vi "fetch_and_translate_trigger.vi"(8 "error in (no error)":errorcluster, 11 "DAQ_DL090211Scaffold in":refnum<class "DAQ_DL090211Scaffold.lvclass">) -> (0 "error out":errorcluster, 1 "sender TLC type":T1=enum."ImagingMode", 2 "trigger":T2, 3 "DAQ_DL090211Scaffold out":refnum<class "DAQ_DL090211Scaffold.lvclass">)   [LabVIEW 2010, in "DAQ_DL090211Scaffold.lvclass"]
uses:
  DAQ_DL090211Scaffold.lvclass
  internal_trigger_enum.ctl
  common/enumerations/top-level_component_type_enum.ctl
  GenericDAQ/GenericDAQ/trigger_enum.ctl
  GenericDAQ/GenericDAQ/GenericDAQ.lvclass
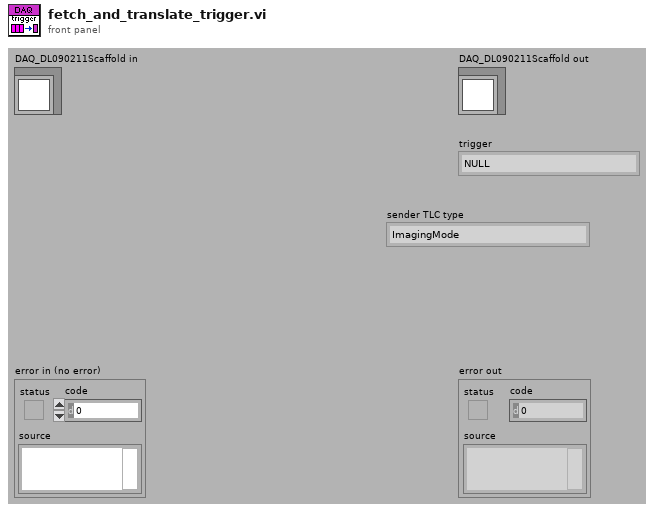
[diagram p1: front panel]
types:
  T1 = typedef "top-level_component_type_enum.ctl" = enum16{"undefined", "ImagingMode", "ScanHead", "DAQ", "ImageAssembler", "Display", "DataCollection", "Analyser", "Stimulator", "ExperimentController", "Instrument", "Stage"}
  T2 = typedef "DAQ_DL090211Scaffold.lvclass/internal_trigger_enum.ctl" = enum16{"NULL", "initialise", "terminate", "start", "stop", "read", "attach observer", "detach observer", "reset"}
  T3 = typedef "GenericDAQ.lvclass/trigger_enum.ctl" = enum16{"NULL", "read"}
  T4 = typedef "GenericToplevelComponent.lvclass/common_trigger_enum.ctl" = enum16{"NULL", "initialise", "terminate", "fetch command", "fetch data", "attach observer", "register as observer", "detach observer", "acknowledge", "start", "stop", "sweep started", "sweep finished", "experiment started", "experiment stopped"}
  T5 = typedef "trigger_type_enum.ctl" = enum8{"external", "internal", "common"}
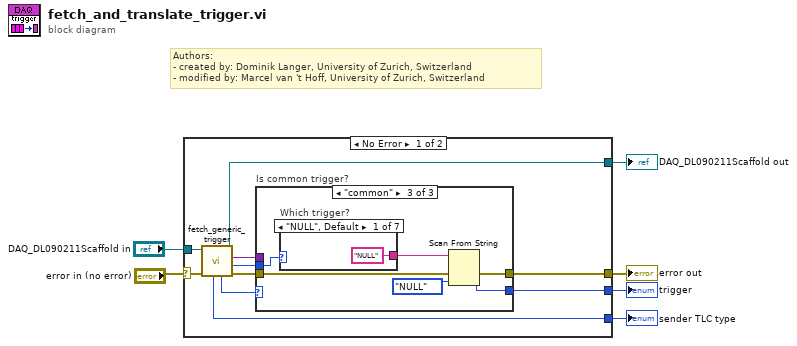
[diagram p0: block diagram]
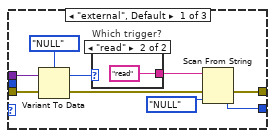
[diagram p2: hidden frame]
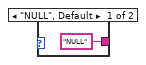
[diagram p3: hidden frame]
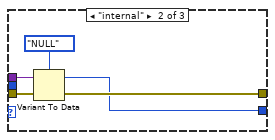
[diagram p4: hidden frame]
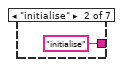
[diagram p5: hidden frame]
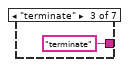
[diagram p6: hidden frame]
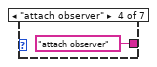
[diagram p7: hidden frame]
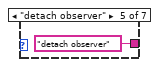
[diagram p8: hidden frame]
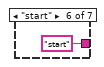
[diagram p9: hidden frame]
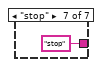
[diagram p10: hidden frame]
diagram:
  # "Authors: \n- created by: Dominik Langer, University of Zurich, Switzerland\n- modified by: Marcel van 't Hoff, University of Zurich, Switzerland"
  n1 = case shown="No Error" "error in (no error)" {
    selector: "error in (no error)" -> [w16 w47]
    tunnel: [w8 w47] -> w5
    tunnel: [w14 w46] -> w3
    tunnel: "DAQ_DL090211Scaffold in" -> [w15 w46]
    tunnel: [w7 _] -> w1
    tunnel: [w9 _] -> w2
    frame No Error {
      n2 = call-dynamic "fetch_generic_trigger.vi"("error in (no error)"=w16, "GenericToplevelComponent in"=w15) -> ("error out"=w12:errorcluster, "common trigger"=w10:T4, "trigger"=w11:variant, "GenericToplevelComponent out"=w14:refnum<class "DAQ_DL090211Scaffold.lvclass">, "trigger type"=w13:T5, "sender TLC type"=w9:T1)  [unwired: 3 in, 1 out]
      n3 = case "Is common trigger?" shown="\"common\"" w13 {
        tunnel: w12 -> [w25 w31 w36]
        tunnel: w11 -> [w24 w32 _]
        tunnel: w10 -> [_ _ w38]
        tunnel: [w20 w29 w33] -> w8
        tunnel: [w17 w28 w34] -> w7
        frame "external", Default {
          n4 = Variant To Data(error in=w25, Variant=w24, type=trigger_enum."NULL" ("message")) -> (error out=w21:errorcluster, data=w22:T3)
          n5 = case "Which trigger?" shown="\"read\"" w22 {
            tunnel: ["NULL" "read"] -> w19
            frame "NULL", Default {
            }
            frame "read" {
            }
          }
          n6 = Scan From String(input string=w19, error in=w21, default 1=internal_trigger_enum."NULL" ("trigger")) -> (error out=w20:errorcluster, output 1=w17:T2)  [unwired: 2 in, 2 out]
        }
        frame "internal" {
          n7 = Variant To Data(error in=w31, Variant=w32, type=internal_trigger_enum."NULL" ("trigger")) -> (error out=w29:errorcluster, data=w28:T2)
        }
        frame "common" {
          n8 = case "Which trigger?" shown="\"NULL\", Default" w38 {
            tunnel: ["NULL" "initialise" "terminate" "attach observer" "detach observer" "start" "stop"] -> w37
            frame "NULL", Default {
            }
            frame "initialise" {
            }
            frame "terminate" {
            }
            frame "attach observer" {
            }
            frame "detach observer" {
            }
            frame "start" {
            }
            frame "stop" {
            }
          }
          n9 = Scan From String(input string=w37, error in=w36, default 1=internal_trigger_enum."NULL" ("trigger")) -> (error out=w33:errorcluster, output 1=w34:T2)  [unwired: 2 in, 2 out]
        }
      }
    }
    frame Error {
    }
  }
  "error out" <- w5
  "DAQ_DL090211Scaffold out" <- w3
  "trigger" <- w1
  "sender TLC type" <- w2
